vi "CheckAlignmentAngles.vi"(9 "Status in":string, 10 "Value":T1) -> (3 "Status out":string)   [LabVIEW 2020]
uses:
  WaferAlignmentType.ctl
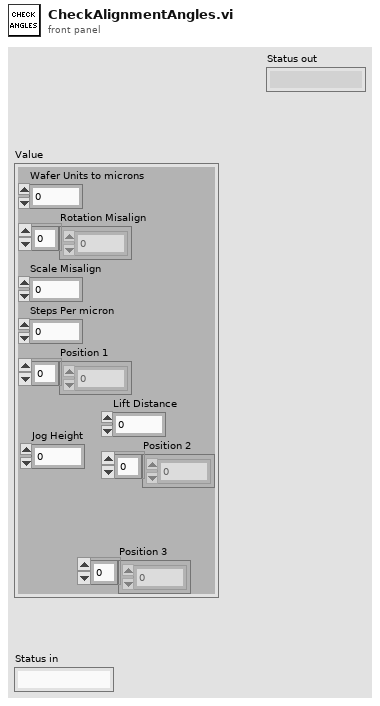
[diagram p1: front panel]
types:
  T1 = typedef "WaferAlignmentType.ctl" = cluster{"Wafer Units to microns":dbl, "Rotation Misalign":dbl[], "Scale Misalign":dbl, "Steps Per micron":dbl, "Position 1":i32[], "Position 2":i32[], "Lift Distance":i32, "Position 3":i32[], "Jog Height":i32}
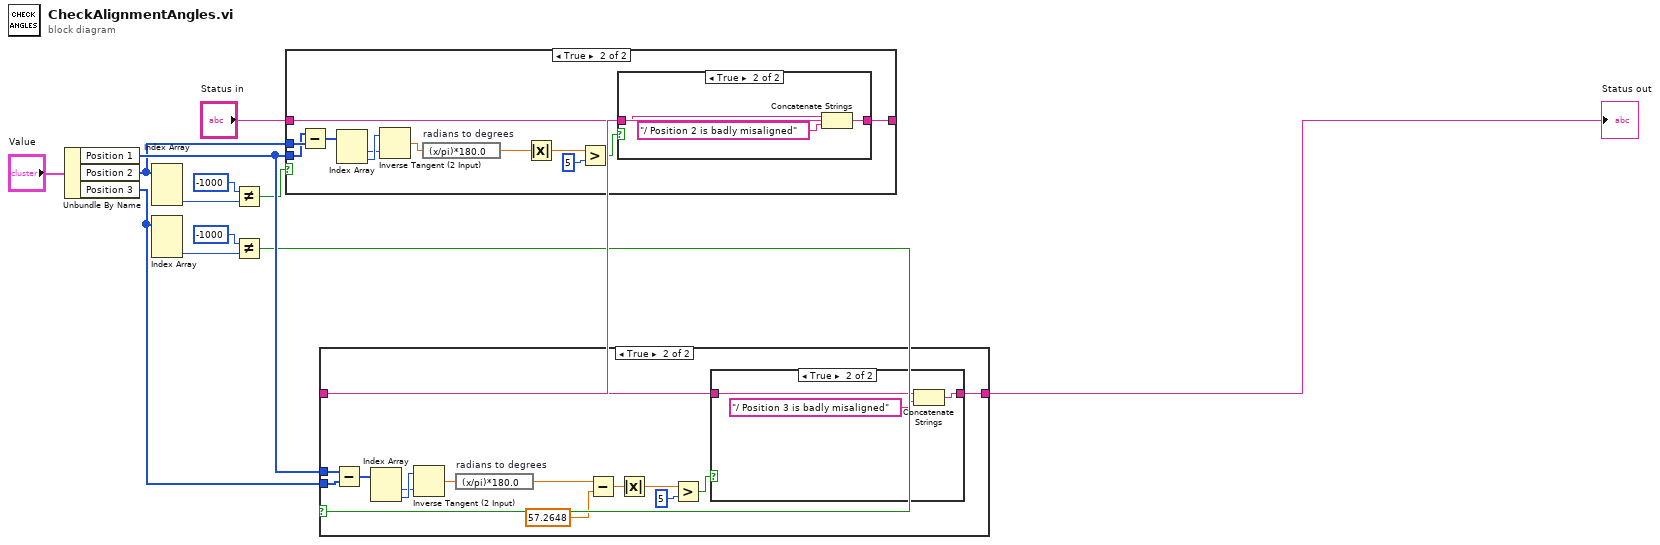
[diagram p0: block diagram]
diagram:
  n1 = Unbundle By Name("Value") -> ("Position 1"=w11:i32[], "Position 2"=w8:i32[], "Position 3"=w2:i32[])
  n2 = Index Array(array=w8) -> (element #3=w7:i32)  [unwired: 3 in, 2 out]
  n3 = Index Array(array=w2) -> (element #3=w4:i32)  [unwired: 3 in, 2 out]
  n4 = Not Equal?(x=-1000, y=w7) -> (x != y?=w5:bool)
  n5 = Not Equal?(x=-1000, y=w4) -> (x != y?=w1:bool)
  n6 = case shown="True" w5 {
    tunnel: "Status in" -> [w14 w26]
    tunnel: w8 -> [_ w23]
    tunnel: w11 -> [_ w22]
    tunnel: [w14 w19] -> w9
    frame False {
    }
    frame True {
      n7 = Subtract(x=w22, y=w23) -> (x-y=w25:i32[])
      n8 = Index Array(array=w25) -> (element #1=w17:i32, element #2=w18:i32)  [unwired: 2 in]
      n9 = Inverse Tangent (2 Input)(1:w17, 2:w18) -> (0:w16:dbl)
      n10 = expression code="(x/pi)*180.0" "radians to degrees"(w16) -> (w15:dbl)
      n11 = Absolute Value(x=w15) -> (abs(x)=w21:dbl)
      n12 = Greater?(x=w21, y=5) -> (0:w24:bool)
      n13 = case shown="True" w24 {
        tunnel: w26 -> [w27 w30]
        tunnel: [w27 w29] -> w19
        frame False {
        }
        frame True {
          n14 = Concatenate Strings(w30, "/ Position 2 is badly misaligned" ("string")) -> (w29:string)
        }
      }
    }
  }
  n15 = case shown="True" w1 {
    tunnel: w2 -> [_ w45]
    tunnel: w11 -> [_ w44]
    tunnel: [w31 w43] -> w10
    tunnel: w9 -> [w31 w42]
    frame False {
    }
    frame True {
      n16 = Subtract(x=w44, y=w45) -> (x-y=w39:i32[])
      n17 = Index Array(array=w39) -> (element #1=w37:i32, element #2=w38:i32)  [unwired: 2 in]
      n18 = Inverse Tangent (2 Input)(1:w37, 2:w38) -> (0:w33:dbl)
      n19 = expression code="(x/pi)*180.0" "radians to degrees"(w33) -> (w32:dbl)
      n20 = Subtract(x=w32, y=57.2648) -> (x-y=w35:dbl)
      n21 = Absolute Value(x=w35) -> (abs(x)=w36:dbl)
      n22 = Greater?(x=w36, y=5) -> (0:w40:bool)
      n23 = case shown="True" w40 {
        tunnel: w42 -> [w46 w49]
        tunnel: [w46 w48] -> w43
        frame False {
        }
        frame True {
          n24 = Concatenate Strings(w49, "/ Position 3 is badly misaligned" ("string")) -> (w48:string)
        }
      }
    }
  }
  "Status out" <- w10
